vi "Generic Check Changes.vi"(10 "New":T1, 11 "Existing":T1) -> (0 "Old Indices":i32[](array[numeric]), 1 "Changed?":bool[](array[boolean]), 2 "Settings":variant[](array[variant]), 3 "Data":variant[](array[variant]))   [LabVIEW 2019, in "Tool Data.lvclass"]
uses:
  Tool Data.lvclass
  Typedefs/Tool Data.Check Changes.ctl
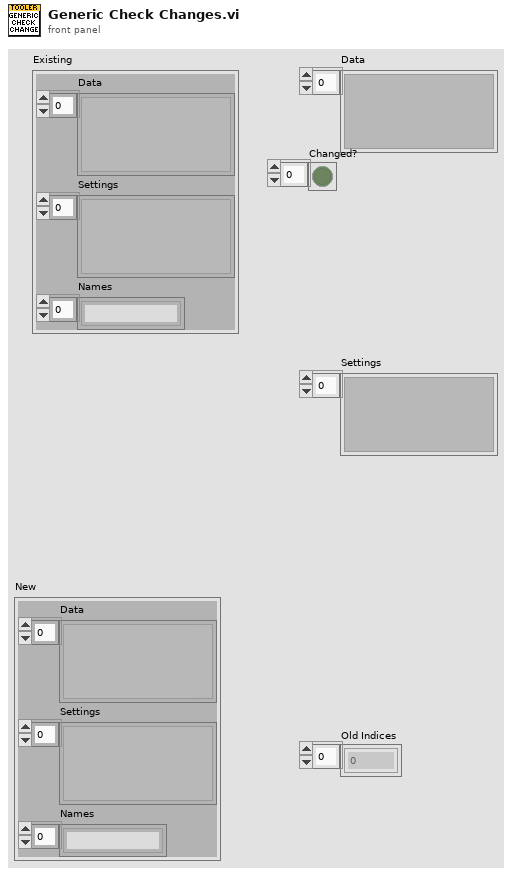
[diagram p1: front panel]
types:
  T1 = typedef "Tool Data.Check Changes.ctl" = cluster{"Data":variant[], "Settings":variant[], "Names":string[]}
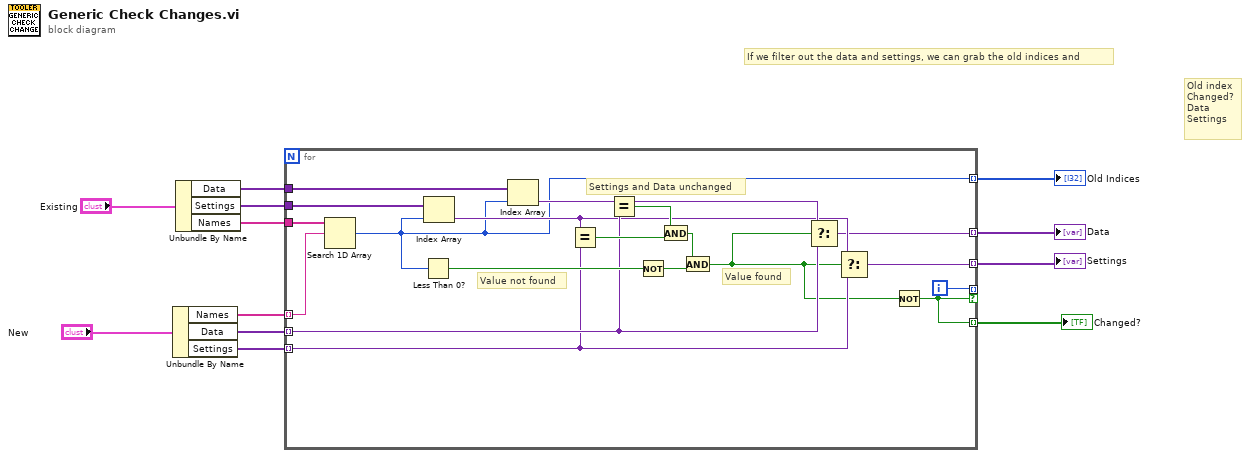
[diagram p0: block diagram]
diagram:
  # "Old index\nChanged?\nData\nSettings"
  # "If we filter out the data and settings, we can grab the old indices and"
  n1 = Unbundle By Name("New") -> ("Names"=w12:string[], "Data"=w11:variant[], "Settings"=w10:variant[])
  n2 = Unbundle By Name("Existing") -> ("Data"=w8:variant[], "Settings"=w7:variant[], "Names"=w6:string[])
  n3 = for {
    tunnel: w6 -> [w31]
    tunnel: w12 -> [w25] mode=indexing
    tunnel: w11 -> [w22] mode=indexing
    tunnel: w10 -> [w20] mode=indexing
    tunnel: w8 -> [w29]
    tunnel: w7 -> [w30]
    tunnel: [w18] -> w4 mode=indexing
    tunnel: [w17] -> w3 mode=indexing
    tunnel: [w16] -> _ mode=indexing if=w13
    tunnel: [w14] -> w5 mode=indexing
    tunnel: [w13] -> w2 mode=indexing
    i -> [w16]
    # "Value found"
    # "Value not found"
    # "Settings and Data unchanged"
    n4 = Search 1D Array(1D array=w31, element=w25) -> (index of element=w14:i32)  [unwired: 1 in]
    n5 = Less Than 0?(x=w14) -> (x < 0?=w24:bool)
    n6 = Index Array(array=w30, index=w14) -> (element=w21:variant)
    n7 = Index Array(array=w29, index=w14) -> (element=w23:variant)
    n8 = Equal?(x=w21, y=w20) -> (x = y?=w27:bool)
    n9 = Equal?(x=w23, y=w22) -> (x = y?=w28:bool)
    n10 = Not(x=w24) -> (.not. x?=w26:bool)
    n11 = And(x=w28, y=w27) -> (x .and. y?=w19:bool)
    n12 = And(x=w19, y=w26) -> (x .and. y?=w15:bool)
    n13 = Select(t=w23, s=w15, f=w22) -> (s? t:f=w18:variant)
    n14 = Select(t=w21, s=w15, f=w20) -> (s? t:f=w17:variant)
    n15 = Not(x=w15) -> (.not. x?=w13:bool)
  }
  "Data" <- w4
  "Settings" <- w3
  "Old Indices" <- w5
  "Changed?" <- w2
